vi "22_ВПГрафикФункции.vi"() -> ()   [LabVIEW 2016]
panel:
  out "Waveform Array":dbl[](array[numeric])
  out "Waveform Graph":cluster{dbl, "Шаг по X":i32, dbl[]}(graph)
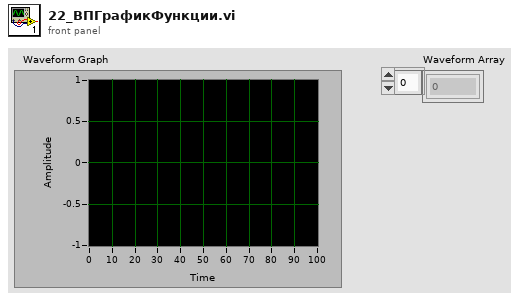
[diagram p1: front panel]
types:
  T1 = cluster{"Начальное X":dbl, "Шаг по X":i32, dbl[]}
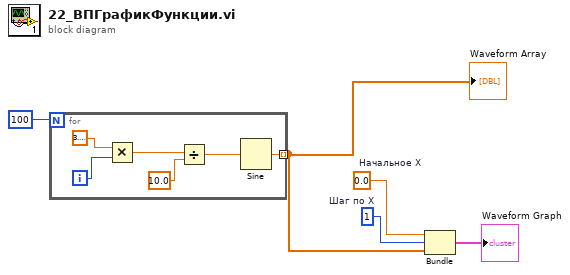
[diagram p0: block diagram]
diagram:
  w3 = 0.0  # Начальное X
  w2 = 1  # Шаг по X
  n1 = for {
    N: 100 -> [_]
    tunnel: [w6] -> w1 mode=indexing
    i -> [w10]
    n2 = Multiply(x=3.141592653589793, y=w10) -> (x*y=w9:dbl)
    n3 = Divide(x=w9, y=10.0) -> (x/y=w7:dbl)
    n4 = Sine(x=w7) -> (sin(x)=w6:dbl)
  }
  "Waveform Array" <- w1
  n5 = Bundle("Начальное X"=w3, "Шаг по X"=w2, w1) -> (→"Waveform Graph":T1)  [unwired: 1 in]
